vi "calculate move to roi.vi"(11 "Coordinates":i32[](array[numeric])) -> (2 "setY":dbl, 3 "setX":dbl)   [LabVIEW 2017]
doc: "SciScan 1.2 160622"
uses:
  GFG/GFGnumericGet.vi
  GFG/GFGbooleanGet.vi
  GFG/GFG library.lvlib
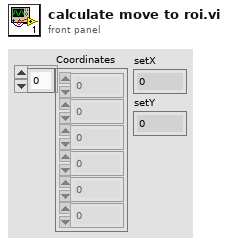
[diagram p1: front panel]
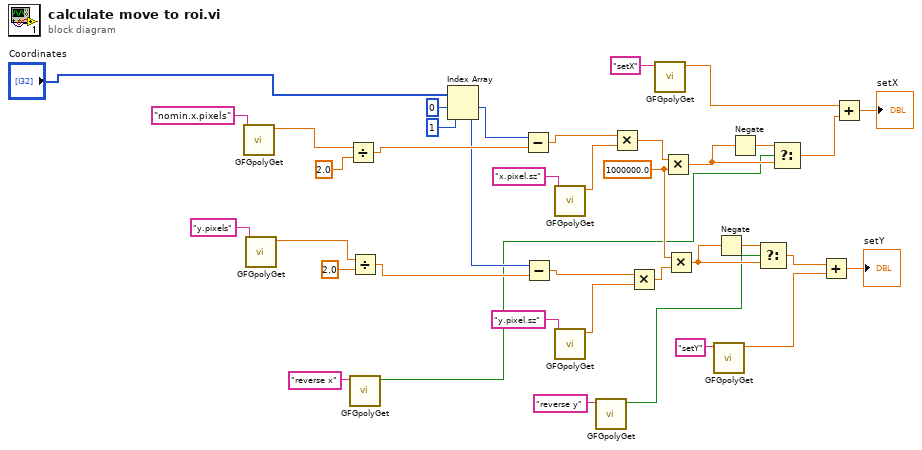
[diagram p0: block diagram]
diagram:
  w15 = 1000000.0 ("y")
  n1 = call-poly "GFGpolyGet.vi"("Variable Name in"="nomin.x.pixels") -> ("Numeric"=w38:dbl)  [unwired: 8 in, 2 out]
  n2 = call-poly "GFGpolyGet.vi"("Variable Name in"="y.pixels") -> ("Numeric"=w33:dbl)  [unwired: 8 in, 2 out]
  n3 = Divide(x=w38, y=2.0) -> (x/y=w28:dbl)
  n4 = Divide(x=w33, y=2.0) -> (x/y=w26:dbl)
  n5 = call-poly "GFGpolyGet.vi"("Variable Name in"="reverse x") -> ("Boolean Value OUT"=w1:bool)  [unwired: 9 in, 1 out]
  n6 = Index Array(array="Coordinates", index #1=0 ("index"), index #2=1 ("index")) -> (element #1=w29:i32, element #2=w27:i32)
  n7 = Subtract(x=w29, y=w28) -> (x-y=w23:dbl)
  n8 = Subtract(x=w27, y=w26) -> (x-y=w21:dbl)
  n9 = call-poly "GFGpolyGet.vi"("Variable Name in"="x.pixel.sz") -> ("Numeric"=w22:dbl)  [unwired: 8 in, 2 out]
  n10 = call-poly "GFGpolyGet.vi"("Variable Name in"="y.pixel.sz") -> ("Numeric"=w20:dbl)  [unwired: 8 in, 2 out]
  n11 = call-poly "GFGpolyGet.vi"("Variable Name in"="reverse y") -> ("Boolean Value OUT"=w3:bool)  [unwired: 9 in, 1 out]
  n12 = Multiply(x=w23, y=w22) -> (x*y=w17:dbl)
  n13 = Multiply(x=w21, y=w20) -> (x*y=w16:dbl)
  n14 = call-poly "GFGpolyGet.vi"("Variable Name in"="setX") -> ("Numeric"=w14:dbl)  [unwired: 8 in, 2 out]
  n15 = Multiply(x=w17, y=w15) -> (x*y=w6:dbl)
  n16 = Multiply(x=w15, y=w16) -> (x*y=w10:dbl)
  n17 = call-poly "GFGpolyGet.vi"("Variable Name in"="setY") -> ("Numeric"=w13:dbl)  [unwired: 8 in, 2 out]
  n18 = Negate(x=w10) -> (-x=w9:dbl)
  n19 = Negate(x=w6) -> (-x=w7:dbl)
  n20 = Select(t=w9, s=w3, f=w10) -> (s? t:f=w8:dbl)
  n21 = Select(t=w7, s=w1, f=w6) -> (s? t:f=w5:dbl)
  n22 = Add(x=w8, y=w13) -> (x+y=→"setY":dbl)
  n23 = Add(x=w14, y=w5) -> (x+y=→"setX":dbl)
